vi "test4.vi"() -> ()   [LabVIEW 2016]
panel:
  out "element":dbl
  out "Array":dbl[](array[numeric])
  out "Numeric 2":i32
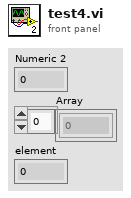
[diagram p1: front panel]
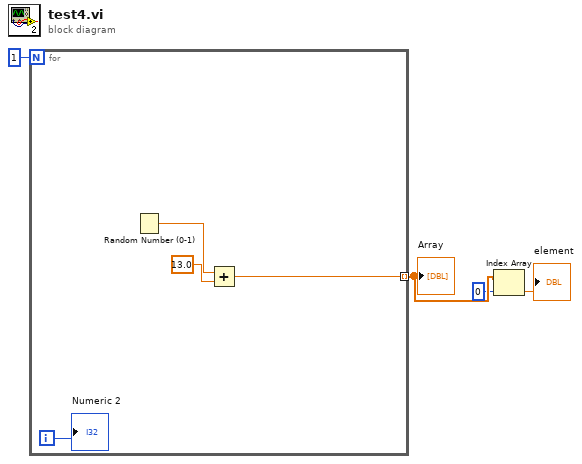
[diagram p0: block diagram]
diagram:
  n1 = for {
    N: 1 -> [_]
    tunnel: [w5] -> w3 mode=indexing
    i -> [w6]
    n2 = Random Number (0-1)() -> (number: 0 to 1=w8:dbl)
    n3 = Add(x=w8, y=13.0) -> (x+y=w5:dbl)
    "Numeric 2" <- w6
  }
  "Array" <- w3
  n4 = Index Array(array=w3, index=0) -> (element=→"element":dbl)
